vi "PipBoy_ReadIconsFile.vi"(8 "error in (no error)":errorcluster, 10 "FileConf":T3) -> (0 "error out":errorcluster, 2 "Icons":T1[](array[typedef]))   [LabVIEW 2014]
uses:
  ctls/PipBoy_FileConf.ctl
  ctls/PipBoy_IconInfo.ctl
  <vilib>/picture/picture.llb/imagedata.ctl
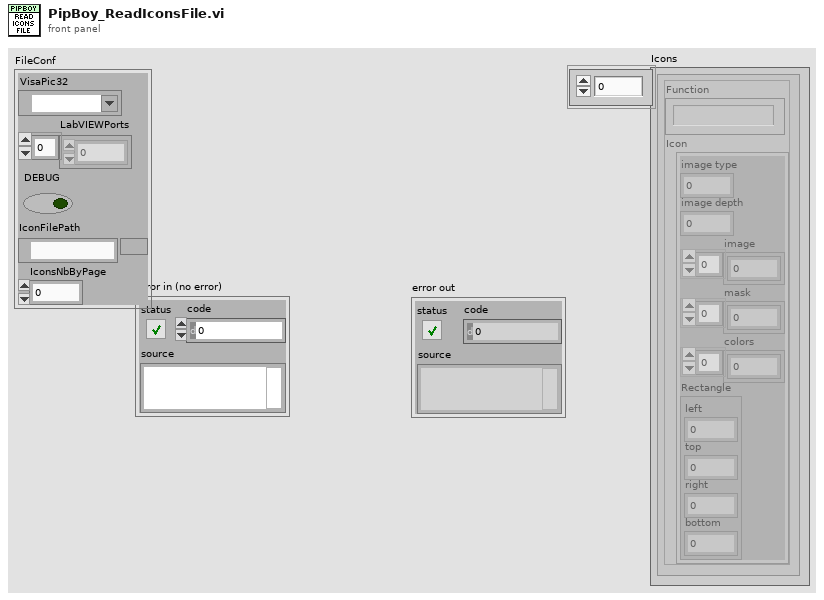
[diagram p1: front panel]
types:
  T1 = typedef "PipBoy_IconInfo.ctl" = cluster{"Function":string, "Icon":T2}
  T2 = typedef "imagedata.ctl" = cluster{"image type":i32, "image depth":i32, "image":u8[], "mask":u8[], "colors":u32[], "Rectangle":cluster{"left":i16, "top":i16, "right":i16, "bottom":i16}}
  T3 = typedef "PipBoy_FileConf.ctl" = cluster{"VisaPic32":refnum<visa-resource-name>, "LabVIEWPorts":u16[], "DEBUG":bool, "IconFilePath":path, "IconsNbByPage":i32}
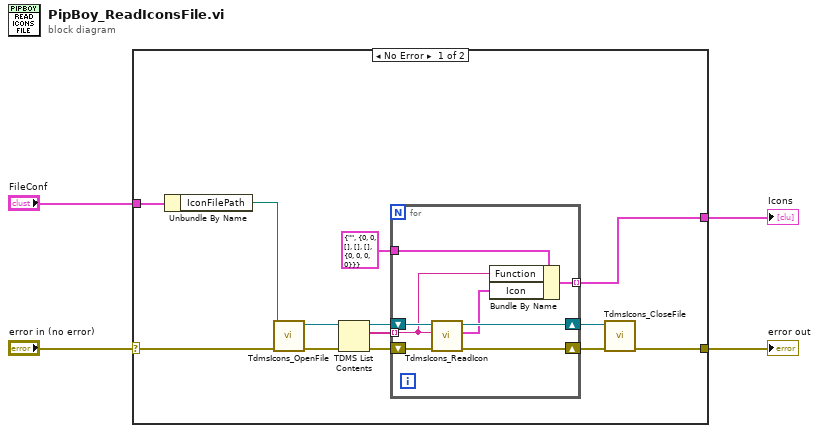
[diagram p0: block diagram]
diagram:
  n1 = case shown="No Error" "error in (no error)" {
    selector: "error in (no error)" -> [w16 w26]
    tunnel: [w7 w26] -> w3
    tunnel: "FileConf" -> [w17 _]
    tunnel: [w5 _] -> w1
    frame No Error {
      n2 = Unbundle By Name(w17) -> ("IconFilePath"=w13:path)
      n3 = call "TdmsIcons_OpenFile.vi"("error in (no error)"=w16, "Path"=w13) -> ("error out"=w15:errorcluster, "TdmsOut"=w14:refnum<k34>)  [unwired: 8 in]
      n4 = TDMS List Contents(4:w15, 7:w14) -> (0:w12:errorcluster, 2:w10:string[], 3:w11:refnum<k34>)  [unwired: 1 in, 1 out]
      n5 = for {
        shift-right: [w23] -> w9
        shift-left: w11 -> [w24]
        tunnel: w10 -> [w19] mode=indexing
        shift-right: [w22] -> w8
        shift-left: w12 -> [w25]
        tunnel: T1 {"Function"="", "Icon"={"image type"=0, "image depth"=0, "image"=[], "mask"=[], "colors"=[], "Rectangle"={"left"=0, "top"=0, "right"=0, "bottom"=0}}} ("Cluster") -> [w21]
        tunnel: [w18] -> w5 mode=indexing
        n6 = call "TdmsIcons_ReadIcon.vi"("error in (no error)"=w25, "Function"=w19, "TdmsIn"=w24) -> ("error out"=w22:errorcluster, "Icon"=w20:T2, "TdmsOut"=w23:refnum<k34>)  [unwired: 6 in]
        n7 = Bundle By Name(cluster=w21, "Function"=w19, "Icon"=w20) -> (w18:T1)
      }
      n8 = call "TdmsIcons_CloseFile.vi"("error in (no error)"=w8, "TdmsIn"=w9) -> ("error out"=w7:errorcluster)  [unwired: 8 in, 1 out]
    }
    frame Error {
    }
  }
  "error out" <- w3
  "Icons" <- w1
